vi "test_word2signal.vi"() -> ()   [LabVIEW 2020]
uses:
  Source/Shared/EncodeDecode/_typedefs/parameter_config_encoding_type.ctl
  Source/Shared/EncodeDecode/_typedefs/parameter_config_type_type.ctl
  Source/Shared/EncodeDecode/_typedefs/parameter_config_type.ctl
panel:
  in  "ParamConfig":T1[](array[typedef])
  in  "words in":u16[](array[numeric]) format="%016b"
  out "parameters out":dbl[](array[numeric])
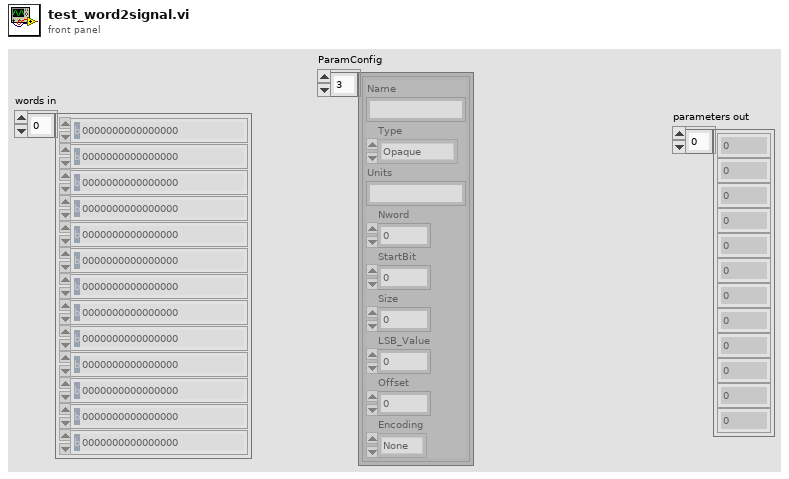
[diagram p1: front panel]
types:
  T1 = typedef "parameter_config_type.ctl" = cluster{"Name":string, "Type":T2, "Units":string, "Nword":i32, "StartBit":i32, "Size":i32, "LSB_Value":i32, "Offset":i32, "Encoding":T3}
  T2 = typedef "parameter_config_type_type.ctl" = enum16{"Opaque", "Enum", "Float", "Integer", "Bcd", "Bool"}
  T3 = typedef "parameter_config_encoding_type.ctl" = enum16{"None", "2-complement", "Unsigned"}
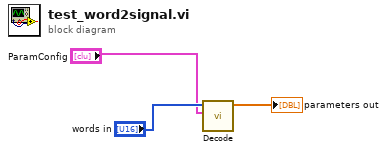
[diagram p0: block diagram]
diagram:
  n1 = call "Decode.vi"("ParamConfig"="ParamConfig", "Words In"="words in") -> ("Parameters out"=→"parameters out":dbl[])  [unwired: 9 in]
